vi "AVT_snap&save_auto.vi"(2 "Save Directory":path, 4 "Filename":string, 7 "CamID":u32=285941632) -> (1 "Image":T1(plugin-control))   [LabVIEW 2015]
doc: "Sample application for controlling AVT cameras.\nPerforms a single-shot via Snap button."
uses:
  <vilib>/vision/NI_Vision_Development_Module.lvlib
panel:
  in  "pnImageHeight":u32=2056
  in  "pnColorCoding":u32
  in  "pnImageWidth":u32=2452
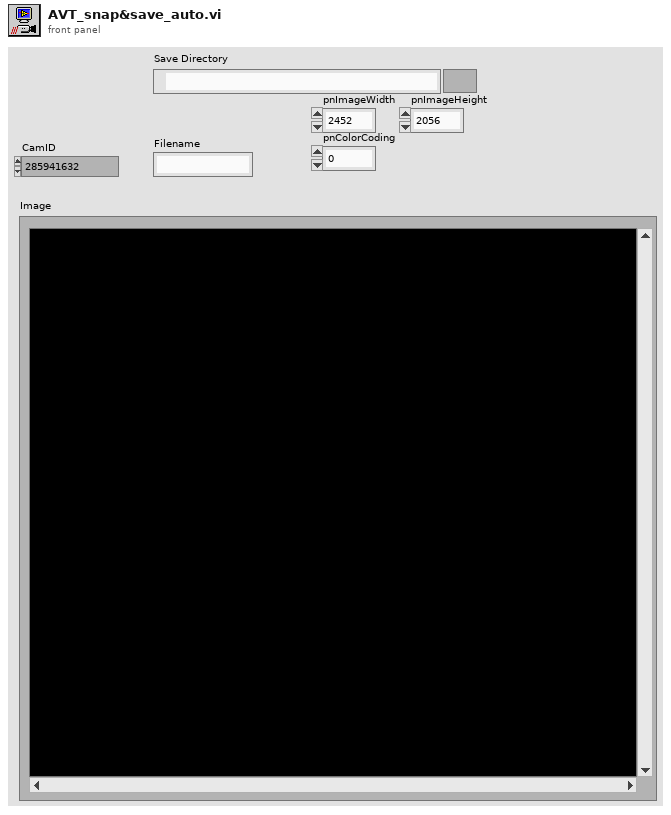
[diagram p1: front panel]
types:
  T1 = typedef "IMAQ Image.ctl" = refnum<image>
  T2 = typedef "Image Type" = u32
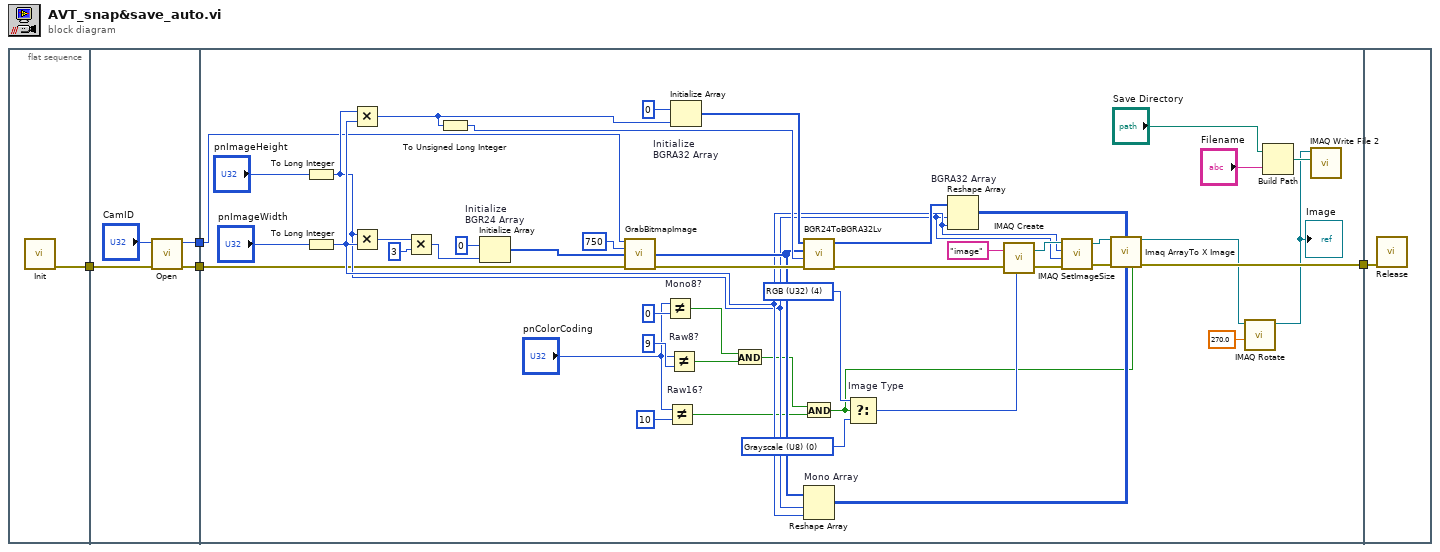
[diagram p0: block diagram]
diagram:
  n1 = flat-sequence {
    tunnel: [w5] -> w3
    tunnel: w3 -> [w9]
    tunnel: [w8] -> w2
    tunnel: [w6] -> w1
    tunnel: w2 -> [w15]
    tunnel: [w19] -> w4
    tunnel: w1 -> [w13]
    tunnel: w4 -> [w56]
    frame #0 {
      n2 = call <userlib>:"Init.vi"() -> ("error out"=w5:errorcluster)  [unwired: 11 out]
    }
    frame #1 {
      n3 = call <userlib>:"Open.vi"("error in (no error)"=w9, "CamId"="CamID") -> ("error out"=w8:errorcluster, "CamId out"=w6:u32)  [unwired: 1 in, 7 out]
    }
    frame #2 {
      w48 = T2 4 items=["Grayscale (U8)", "Grayscale (I16)", "Grayscale (SGL)", "Complex (CSG)", "RGB (U32)", "HSL (U32)", "RGB (U64)"] ("Image Type")
      w47 = T2 0 items=["Grayscale (U8)", "Grayscale (I16)", "Grayscale (SGL)", "Complex (CSG)", "RGB (U32)", "HSL (U32)", "RGB (U64)"] ("Image Type")
      n4 = To Long Integer(number="pnImageHeight") -> (32bit integer=w30:i32)
      n5 = To Long Integer(number="pnImageWidth") -> (32bit integer=w31:i32)
      n6 = Multiply(x=w30, y=w31) -> (x*y=w36:i32)
      n7 = Multiply(x=w30, y=w31) -> (x*y=w52:i32)
      n8 = Multiply(x=w52, y=3) -> (x*y=w35:i32)
      n9 = To Unsigned Long Integer(number=w36) -> (unsigned 32bit integer=w40:u32)
      n10 = Initialize Array "Initialize\nBGR24 Array"(u8 0 ("element"), w35) -> (w33:u8[])
      n11 = call <userlib>:"GrabBitmapImage.vi"("CamId"=w13, "nTimeOut"=u32 750, "pImage In"=w33, "error in (no error)"=w15) -> ("pImage"=w34:u8[], "error out"=w38:errorcluster)  [unwired: 1 in, 9 out]
      n12 = Not Equal? "Mono8?"(x="pnColorCoding", y=u32 0) -> (x != y?=w24:bool)
      n13 = Not Equal? "Raw16?"(x="pnColorCoding", y=u32 10) -> (x != y?=w26:bool)
      n14 = Not Equal? "Raw8?"(x="pnColorCoding", y=u32 9) -> (x != y?=w25:bool)
      n15 = Initialize Array "Initialize\nBGRA32 Array"(u32 0 ("element"), w36) -> (w41:u32[])
      n16 = And(x=w24, y=w25) -> (x .and. y?=w23:bool)
      n17 = call <userlib>:"BGR24ToBGRA32Lv.vi"("error in (no error)"=w38, "nPixelCount"=w40, "pSrc"=w34, "pDst In"=w41) -> ("error out"=w37:errorcluster, "pDst"=w39:u32[])  [unwired: 6 out]
      n18 = And(x=w23, y=w26) -> (x .and. y?=w22:bool)
      n19 = Reshape Array "Mono Array"(w34, w30, w31) -> (w44:u8[][])
      n20 = Select "Image Type"(t=w48, s=w22, f=w47) -> (s? t:f=w46:T2)
      n21 = Reshape Array "BGRA32 Array"(w39, w30, w31) -> (w49:u32[][])
      n22 = call "IMAQ Create"("Image Name"="image", "Image Type"=w46, "error in (no error)"=w37) -> ("New Image"=w54:T1, "error out"=w55:errorcluster)  [unwired: 1 in, 1 out]
      n23 = call "IMAQ SetImageSize"("error in (no error)"=w55, "Y Resolution"=w30, "X Resolution"=w31, "Image"=w54) -> ("error out"=w43:errorcluster, "Image Out"=w42:T1)  [unwired: 1 out]
      n24 = call <userlib>:"Imaq ArrayTo X Image.vi"("Image"=w42, "Image Pixels (U32)"=w49, "error in (no error)"=w43, "Image Pixels (U8)"=w44, "IsColor"=w22) -> ("Image Out"=w12:T1, "error out"=w19:errorcluster)  [unwired: 9 out]
      n25 = call "IMAQ Rotate"("Angle (degrees)"=sgl 270.0, "Image Src"=w12) -> ("Image Dst Out"=w11:T1)  [unwired: 8 in, 1 out]
      "Image" <- w11
      n26 = Build Path(base path="Save Directory", name or relative path="Filename") -> (appended path=w17:path)
      n27 = call-poly "IMAQ Write File 2"("File Path"=w17, "Image"=w11) -> ()  [unwired: 8 in, 2 out]
    }
    frame #3 {
      n28 = call <userlib>:"Release.vi"("error in (no error)"=w56) -> ()  [unwired: 11 out]
    }
  }
